vi "img_make_1ea-2.vi"() -> ()   [LabVIEW 2016]
uses:
  <vilib>/Utility/file.llb/Write Delimited Spreadsheet (I64).vi
  <vilib>/vision/NI_Vision_Development_Module.lvlib
panel:
  in  "fname":string="lego"
  out "크기":i32[](array[numeric])=[28, 28]
  in  "fpath_jpg":path=path "C:/Users/NB-SH-001/Documents/Python Scripts/data/img_small/07_lego/lego_img"
  in  "fpath_txt":path=path "C:/Users/NB-SH-001/Documents/Python Scripts/data/img_small/07_lego/lego_txt"
  in  "yoffsetscale":dbl=8.0 format="%#_13g"
  in  "xoffsetscale":dbl=8.0 format="%#_13g"
  in  "X Resolution":i32=28
  in  "Y Resolution":i32=28
  out "count":i32=360
  out "Image Pixels (U8)":u8[][](array[numeric])
  out "Image 3":T1(plugin-control)
  in  "Angle (degrees)":sgl=87.0 format="%.2f"
  in  "정지":bool
  in  "X Step Size":i32=1
  in  "Y Step Size":i32=1
  in  "Optional Rectangle":i32[](array[numeric])=[50, 57, 327, 268]
  out "Image 2":T1(plugin-control)
  out "Image":T1(plugin-control)
  in  "fpath_ori_jpg":path=path "C:/Users/NB-SH-001/Documents/Python Scripts/data/img/Classification/Legos01.jpg"
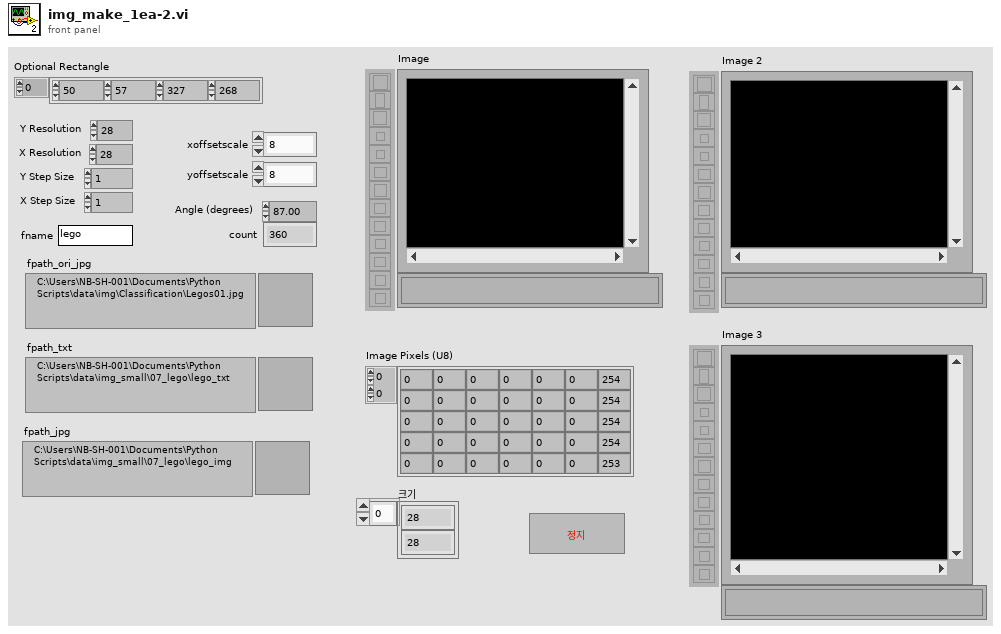
[diagram p1: front panel]
types:
  T1 = typedef "IMAQ Image.ctl" = refnum<image>
  T2 = typedef "Image Type" = u32
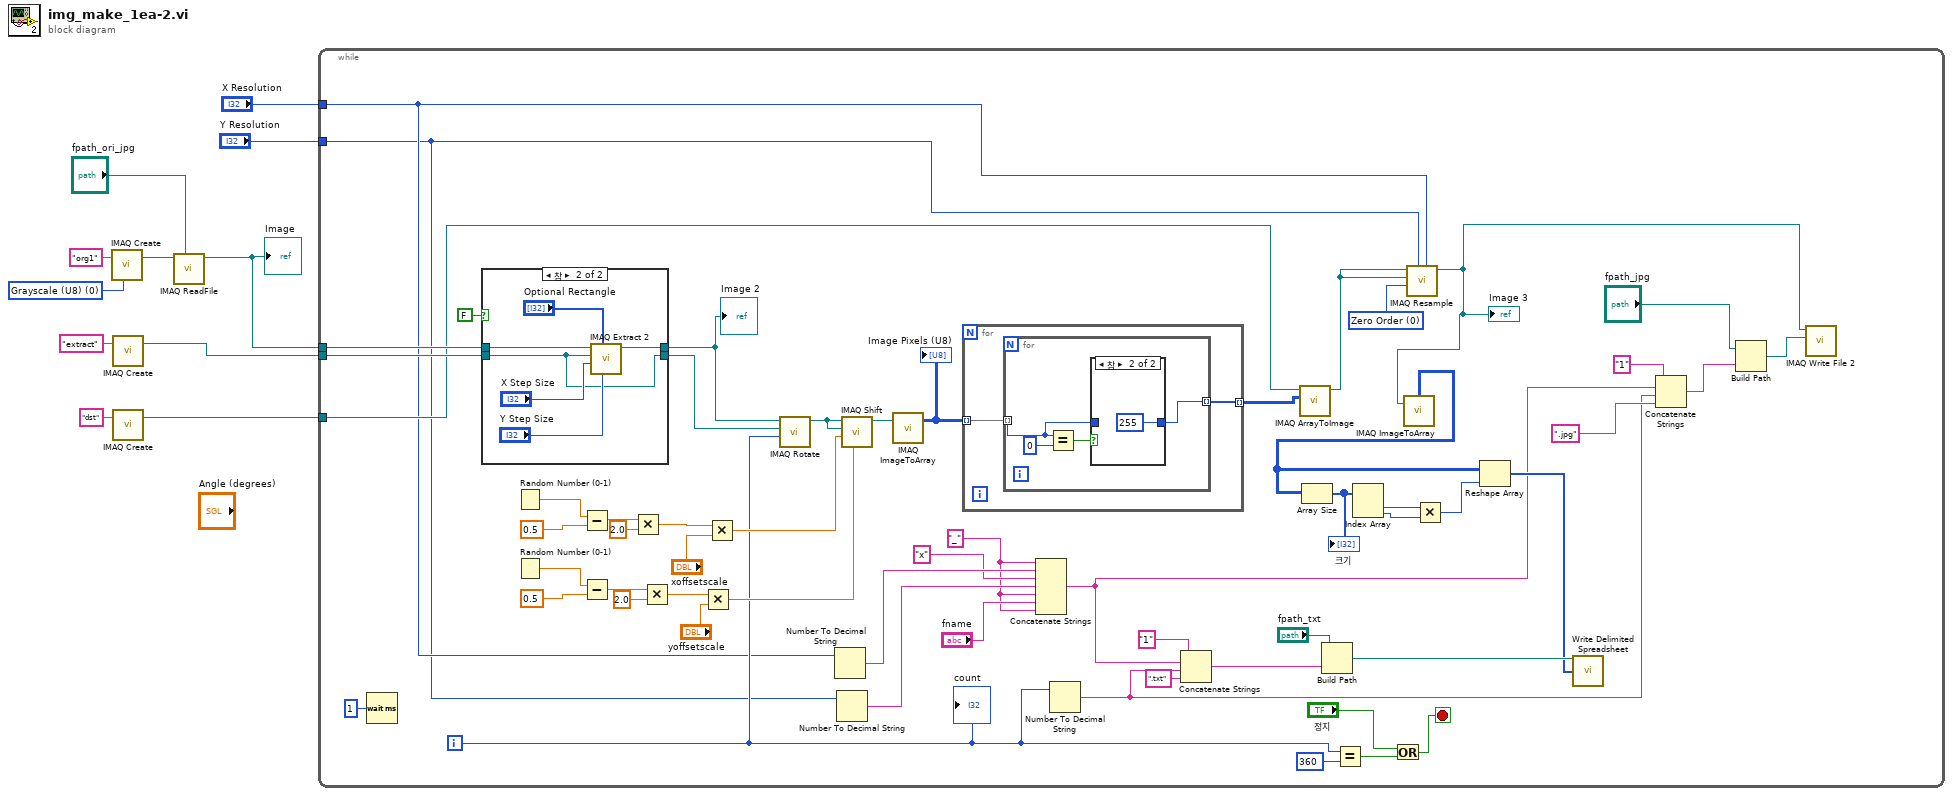
[diagram p0: block diagram]
diagram:
  w3 = T2 0 items=["Grayscale (U8)", "Grayscale (I16)", "Grayscale (SGL)", "Complex (CSG)", "RGB (U32)", "HSL (U32)", "RGB (U64)", "Grayscale (U16)"] ("Image Type")
  n1 = call "IMAQ Create"("Image Name"="org1", "Image Type"=w3) -> ("New Image"=w10:T1)  [unwired: 3 in, 1 out]
  n2 = call "IMAQ Create"("Image Name"="extract") -> ("New Image"=w6:T1)  [unwired: 4 in, 1 out]
  n3 = call "IMAQ Create"("Image Name"="dst") -> ("New Image"=w4:T1)  [unwired: 4 in, 1 out]
  n4 = call "IMAQ ReadFile"("File Path"="fpath_ori_jpg", "Image"=w10) -> ("Image Out"=w7:T1)  [unwired: 5 in, 4 out]
  "Image" <- w7
  n5 = while {
    tunnel: w7 -> [w69]
    tunnel: w6 -> [w68]
    tunnel: w4 -> [w64]
    tunnel: "X Resolution" -> [w19]
    tunnel: "Y Resolution" -> [w18]
    i -> [w35]
    stop <- w52 stop-if-true
    w13 = "_" ("문자열")
    w41 = u32 0 items=["Zero Order", "Bi-Linear", "Quadratic", "Cubic Spline"] ("Interpolation Type")
    n6 = Wait (ms)(milliseconds to wait=u32 1 ("대기 시간 (ms)")) -> ()  [unwired: 1 out]
    n7 = case shown="참" FALSE {
      tunnel: w69 -> [w71 w77]
      tunnel: w68 -> [w70 w72]
      tunnel: [w71 w73] -> w66
      tunnel: [w70 w72] -> w60
      frame False {
      }
      frame True {
        n8 = call "IMAQ Extract 2"("Y Step Size"="Y Step Size", "Optional Rectangle"="Optional Rectangle", "X Step Size"="X Step Size", "Image Dst"=w72, "Image Src"=w77) -> ("Image Dst Out"=w73:T1)  [unwired: 5 in, 1 out]
      }
    }
    "Image 2" <- w66
    n9 = Random Number (0-1)() -> (number: 0 to 1=w59:dbl)
    n10 = Random Number (0-1)() -> (number: 0 to 1=w56:dbl)
    n11 = Subtract(x=w59, y=0.5) -> (x-y=w51:dbl)
    n12 = Subtract(x=w56, y=0.5) -> (x-y=w48:dbl)
    n13 = Multiply(x=w51, y=2.0) -> (x*y=w46:dbl)
    n14 = Multiply(x=w48, y=2.0) -> (x*y=w44:dbl)
    n15 = Multiply(x=w44, y="yoffsetscale") -> (x*y=w42:dbl)
    n16 = Multiply(x=w46, y="xoffsetscale") -> (x*y=w43:dbl)
    n17 = call "IMAQ Rotate"("Angle (degrees)"=w35, "Image Dst"=w60, "Image Src"=w66) -> ("Image Dst Out"=w63:T1)  [unwired: 7 in, 1 out]
    n18 = Number To Decimal String(number=w19) -> (decimal integer string=w17:string)  [unwired: 1 in]
    n19 = Number To Decimal String(number=w18) -> (decimal integer string=w15:string)  [unwired: 1 in]
    n20 = call "IMAQ Shift"("YOffset"=w42, "XOffset"=w43, "Image Dst"=w63, "Image Src"=w63) -> ("Image Dst Out"=w62:T1)  [unwired: 6 in, 1 out]
    n21 = call "IMAQ ImageToArray"("Image"=w62) -> ("Image Pixels (U8)"=w65:u8[][])  [unwired: 3 in, 4 out]
    "Image Pixels (U8)" <- w65
    n22 = for {
      tunnel: w65 -> [w79] mode=indexing
      tunnel: [w78] -> w21 mode=indexing
      n23 = for {
        tunnel: w79 -> [w81] mode=indexing
        tunnel: [w80] -> w78 mode=indexing
        n24 = Equal?(x=w81, y=u8 0) -> (x = y?=w82:bool)
        n25 = case shown="참" w82 {
          tunnel: [w84 u8 255] -> w80
          tunnel: w81 -> [w84 _]
          frame False {
          }
          frame True {
          }
        }
      }
    }
    n26 = Concatenate Strings(w13, w17, "x" ("문자열"), w15, w13, "fname", w13) -> (w12:string)
    n27 = Number To Decimal String(number=w35) -> (decimal integer string=w26:string)  [unwired: 1 in]
    n28 = Concatenate Strings("1" ("문자열"), w12, w26, ".txt" ("문자열")) -> (w38:string)
    n29 = call "IMAQ ArrayToImage"("Image Pixels (U8)"=w21, "Image"=w64) -> ("Image Out"=w40:T1)  [unwired: 8 in, 1 out]
    n30 = Build Path(base path="fpath_txt", name or relative path=w38) -> (appended path=w37:path)
    n31 = Equal?(x=w35, y=360) -> (x = y?=w54:bool)
    n32 = Or(x="정지", y=w54) -> (x .or. y?=w52:bool)
    n33 = call "IMAQ Resample"("X Resolution"=w19, "Y Resolution"=w18, "Interpolation Type"=w41, "Image Dst"=w40, "Image Src"=w40) -> ("Image Dst Out"=w22:T1)  [unwired: 5 in, 1 out]
    "Image 3" <- w22
    n34 = call "IMAQ ImageToArray"("Image"=w22) -> ("Image Pixels (U8)"=w20:u8[][])  [unwired: 3 in, 4 out]
    n35 = Array Size(array=w20) -> (size(s)=w32:i32[])
    "크기" <- w32
    n36 = Index Array(array=w32) -> (element #1=w30:i32, element #2=w31:i32)  [unwired: 2 in]
    n37 = Multiply(x=w30, y=w31) -> (x*y=w33:i32)
    n38 = Reshape Array(w20, w33) -> (w23:u8[])
    n39 = call-poly <vilib>:"Write Delimited Spreadsheet.vi"("file path (dialog if empty)"=w37, "1D data"=w23) -> ()  [unwired: 12 in, 2 out]
    n40 = Concatenate Strings("1" ("문자열"), w12, w26, ".jpg" ("문자열")) -> (w28:string)
    n41 = Build Path(base path="fpath_jpg", name or relative path=w28) -> (appended path=w24:path)
    n42 = call-poly "IMAQ Write File 2"("File Path"=w24, "Image"=w22) -> ()  [unwired: 8 in, 2 out]
    "count" <- w35
  }
